vi "Is Cluster Wire.vi"(8 "error in":errorcluster, 10 "User VI Ref":refnum<vi>, 11 "Affected Items":T1) -> (0 "error out":errorcluster, 1 "Data Type":variant, 2 "Refnum Wire?":bool, 3 "Cluster Wire?":bool)   [LabVIEW 2023]
doc: "Determine if the selected wire carries a cluster value, and return a reference to the cluster itself for later use.\n\nOr determines if wire is a refnum wire and returns a reference to its data type.\n\nAlso checks to see if only one wire is selected."
uses:
  top/BundleMagic.ctl
  <vilib>/Utility/Data Type/NI_Data Type.lvlib
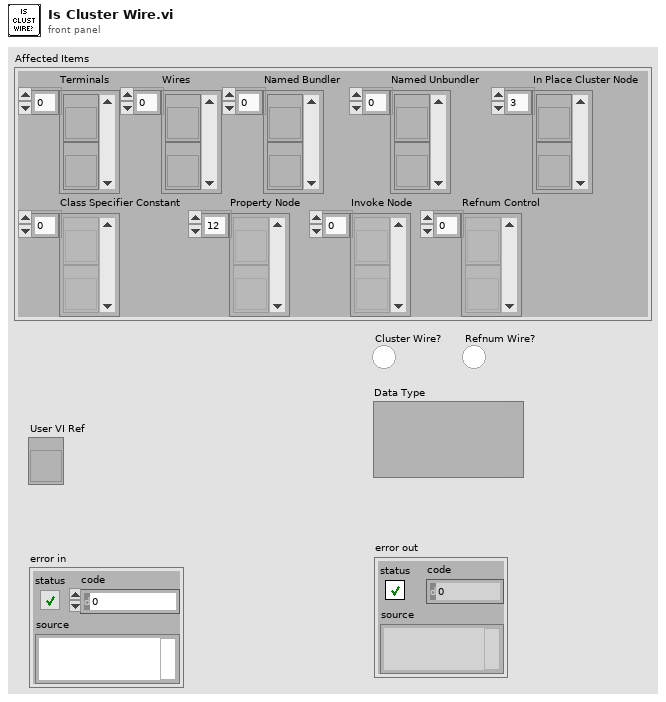
[diagram p1: front panel]
types:
  T1 = typedef "BundleMagic.ctl" = cluster{"Terminals":refnum<vi>[], "Wires":refnum<vi>[], "Named Bundler":refnum<vi>[], "Named Unbundler":refnum<vi>[], "In Place Cluster Node":refnum<vi>[], "Class Specifier Constant":refnum<vi>[], "Property Node":refnum<vi>[], "Invoke Node":refnum<vi>[], "Refnum Control":refnum<vi>[]}
  T2 = typedef "NI_Data Type.lvlib/Data Type.ctl" = enum8{"Invalid Type", "Void", "I8", "I16", "I32", "I64", "U8", "U16", "U32", "U64", "Single Float", "Double Float", "Extended Float", "Single Complex", "Double Complex", "Extended Complex", "Enum U8", "Enum U16", "Enum U32", "Enum U64", "Single Float With Unit", "Double Float With Unit", "Extended Float With Unit", "Single Complex with Unit", "Double Complex with Unit", "Extended Complex with Unit", "Boolean", "String", "Path", "Picture", "Tag", "Array", "Cluster", "Variant", "LV Variant", "Waveform", "Timestamp", "Digital Waveform", "Digital Data", "ExpressData", "Refnum", "External Data", "VI", "Poly VI", "LabVIEW Class Instance", "Fixed Point", "Set Collection", "Map Collection"}
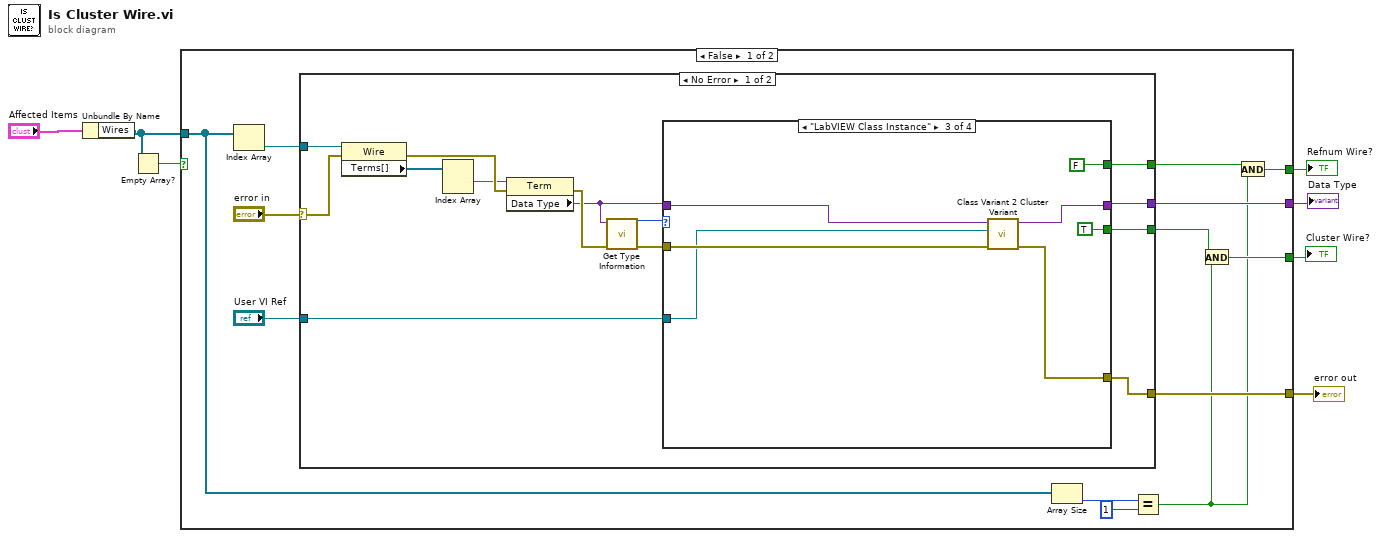
[diagram p0: block diagram]
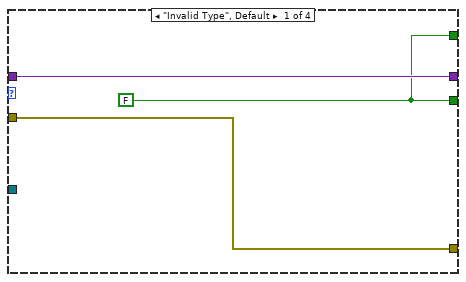
[diagram p2: hidden frame]
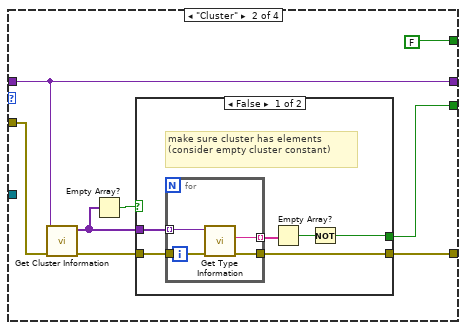
[diagram p3: hidden frame]
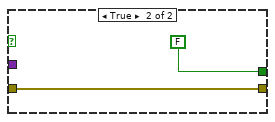
[diagram p4: hidden frame]
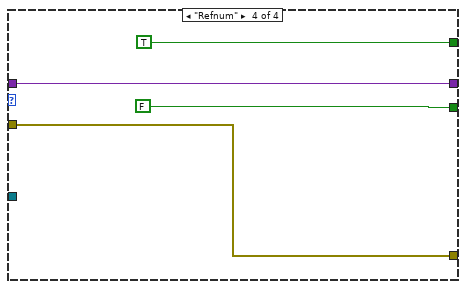
[diagram p5: hidden frame]
diagram:
  n1 = Unbundle By Name("Affected Items") -> ("Wires"=w6:refnum<vi>[])
  n2 = Empty Array?(array=w6) -> (empty?=w5:bool)
  n3 = case shown="False" w5 {
    tunnel: w6 -> [w14 _]
    tunnel: [w13 _] -> w4
    tunnel: [w12 _] -> w3
    tunnel: [w11 _] -> w2
    tunnel: [w8 _] -> w1
    frame False {
      n4 = Index Array(array=w14) -> (element=w15:refnum<vi>)  [unwired: 1 in]
      n5 = case shown="No Error" "error in" {
        selector: "error in" -> [w33 w69]
        tunnel: [w30 _] -> w13
        tunnel: [w25 w69] -> w11
        tunnel: [w29 _] -> w16
        tunnel: "User VI Ref" -> [w24 _]
        tunnel: w15 -> [w22 _]
        tunnel: [w21 _] -> w10
        frame No Error {
          n6 = property class="Wire"(reference=w22, error in=w33) -> (error out=w34:errorcluster, "Terms[]"=w26:refnum<vi>[])  [unwired: 1 out]
          n7 = Index Array(array=w26) -> (element #1=w23:refnum<vi>)  [unwired: 2 in, 1 out]
          n8 = property class="Term"(reference=w23, error in=w34) -> (error out=w28:errorcluster, "Data Type"=w27:variant)  [unwired: 1 out]
          n9 = call <vilib>:"Get Type Information.vi"("error in (no error)"=w28, "variant"=w27) -> ("error out"=w31:errorcluster, "type"=w32:T2)  [unwired: 5 in, 3 out]
          n10 = case shown="\"LabVIEW Class Instance\"" w32 {
            tunnel: w27 -> [w36 w38 w64 w66]
            tunnel: [w37 w41 w62 w65] -> w25
            tunnel: w31 -> [w37 w40 w63 w65]
            tunnel: [w36 w38 w60 w66] -> w30
            tunnel: [w35 w39 TRUE FALSE] -> w29
            tunnel: w24 -> [_ _ w59 _]
            tunnel: [w35 FALSE FALSE TRUE] -> w21
            frame "Invalid Type", Default {
              w35 = FALSE
            }
            frame "Cluster" {
              n11 = call <vilib>:"Get Cluster Information.vi"("error in (no error)"=w40, "variant"=w38) -> ("error out"=w42:errorcluster, "cluster elements"=w43:variant[])  [unwired: 8 in]
              n12 = Empty Array?(array=w43) -> (empty?=w44:bool)
              n13 = case shown="False" w44 {
                tunnel: w43 -> [w51 _]
                tunnel: [w48 FALSE] -> w39
                tunnel: w42 -> [w47 w56]
                tunnel: [w46 w56] -> w41
                frame False {
                  # "make sure cluster has elements (consider empty cluster constant)"
                  n14 = for {
                    tunnel: w51 -> [w55] mode=indexing
                    tunnel: [w54] -> w50 mode=indexing
                    tunnel: w47 -> [w53]
                    tunnel: [w52] -> w46
                    n15 = call <vilib>:"Get Type Information.vi"("error in (no error)"=w53, "variant"=w55) -> ("error out"=w52:errorcluster, "name"=w54:string)  [unwired: 5 in, 3 out]
                  }
                  n16 = Empty Array?(array=w50) -> (empty?=w49:bool)
                  n17 = Not(x=w49) -> (.not. x?=w48:bool)
                }
                frame True {
                }
              }
            }
            frame "LabVIEW Class Instance" {
              n18 = call "Class Variant 2 Cluster Variant.vi"("error in (no error)"=w63, "User VI Ref"=w59, "Variant"=w64) -> ("error out"=w62:errorcluster, "Control Value:Get"=w60:variant)  [unwired: 7 in]
            }
            frame "Refnum" {
            }
          }
        }
        frame Error {
        }
      }
      n19 = Array Size(array=w14) -> (size(s)=w17:i32)
      n20 = Equal?(x=w17, y=1) -> (x = y?=w9:bool)
      n21 = And(x=w16, y=w9) -> (x .and. y?=w12:bool)
      n22 = And(x=w10, y=w9) -> (x .and. y?=w8:bool)
    }
    frame True {
    }
  }
  "Data Type" <- w4
  "Cluster Wire?" <- w3
  "error out" <- w2
  "Refnum Wire?" <- w1
